vi "Window_plot.vi"() -> ()   [LabVIEW 2022 SP3]
doc: "This window has the capability to visualize and analyze the graphs of the stored signals from the Main_menu."
uses:
  <vilib>/Waveform/WDTOps.llb/WDT Get Waveform Subset DBL.vi
panel:
  in  "Slide Offset":u32(slide) scale=0.0..10.0
  in  "Select offset":string(combo)
  out "Waveform Graph":waveform(dbl)[](graph) caption="Waveform Graph 2"
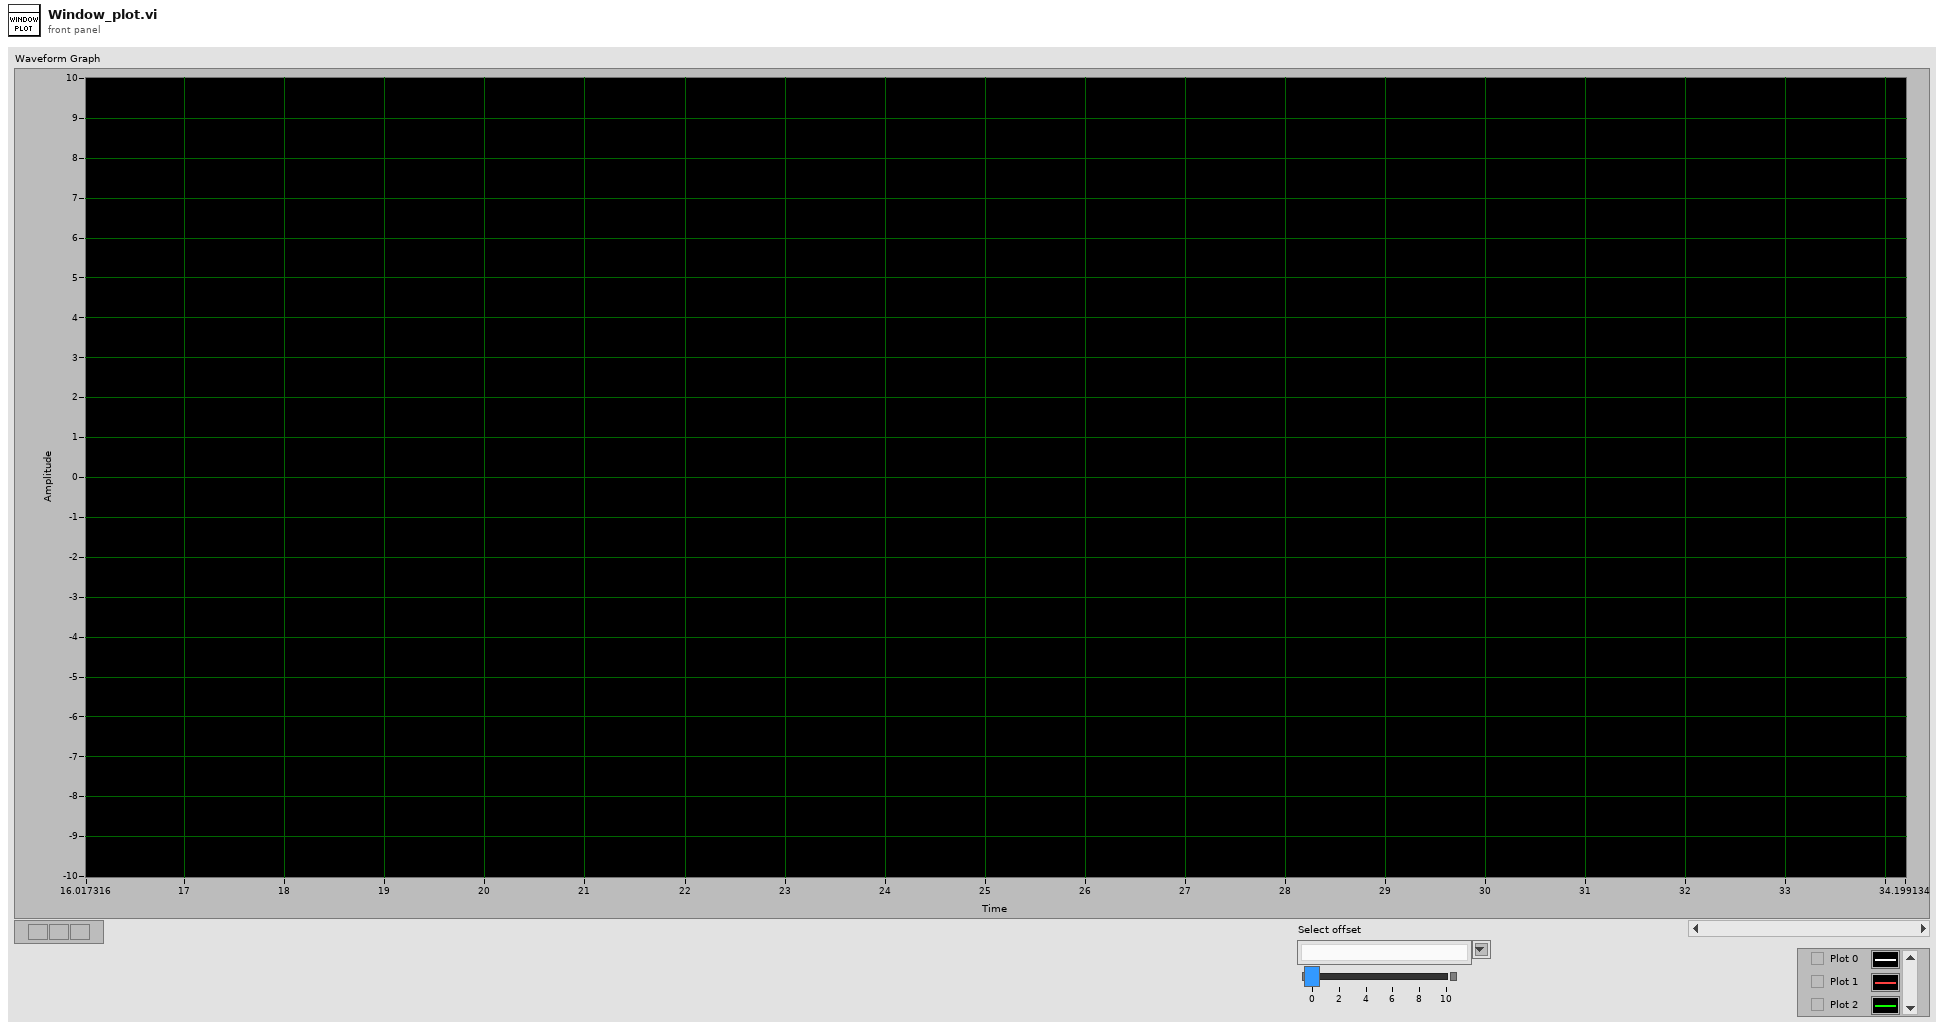
[diagram p1: front panel]
types:
  T1 = cluster{"Mode signal_Global":refnum<vi>, "Trace name":refnum<vi>, "Execution:State":refnum<vi>, "message":refnum<vi>, "Filename":refnum<vi>, "Closed w":refnum<vi>, "total \nrefresh time":refnum<vi>, "Mode signal_Global 2":string, "Filename 2":string, "Execution:State 2":enum32{"Bad", "Idle", "Run top level", "Running"}, "message 2":string, "Trace name 2":string, "total \nrefresh time 2":i32, "refresh time 2":i32, "Continous":bool}
  T2 = cluster{"plot Names":string[], "Waveforms arrays":waveform(dbl)[], "signals_HW":string[][], "Waveforms arrays csv":waveform(dbl)[], "signals_csv":string[], "Signals_name":string[], "Mode_signal_conf":u8, "Request_plots_array":cluster{string, waveform(dbl)}[], "time out":i32, " global r time":u32, "Refresh time":u32, "Local Mode":enum32{"Resume", "Hold"}}
  T3 = enum32{"Invalid", "Standard", "Closed", "Hidden", "Minimized", "Maximized"}
  T4 = enum32{"Bad", "Idle", "Run top level", "Running"}
  T5 = cluster{"plot Names":string[], "Waveforms arrays":waveform(dbl)[], "signals_HW":string[][], "Waveforms arrays csv":waveform(dbl)[], "signals_csv":string[], "Signals_name":string[], "Mode_signal_conf":u8, "Request_plots_array":cluster{string, "Waveform":waveform(dbl)}[], "time out":i32, " global r time":u32, "Refresh time":u32, "Local Mode":enum32{"Resume", "Hold"}}
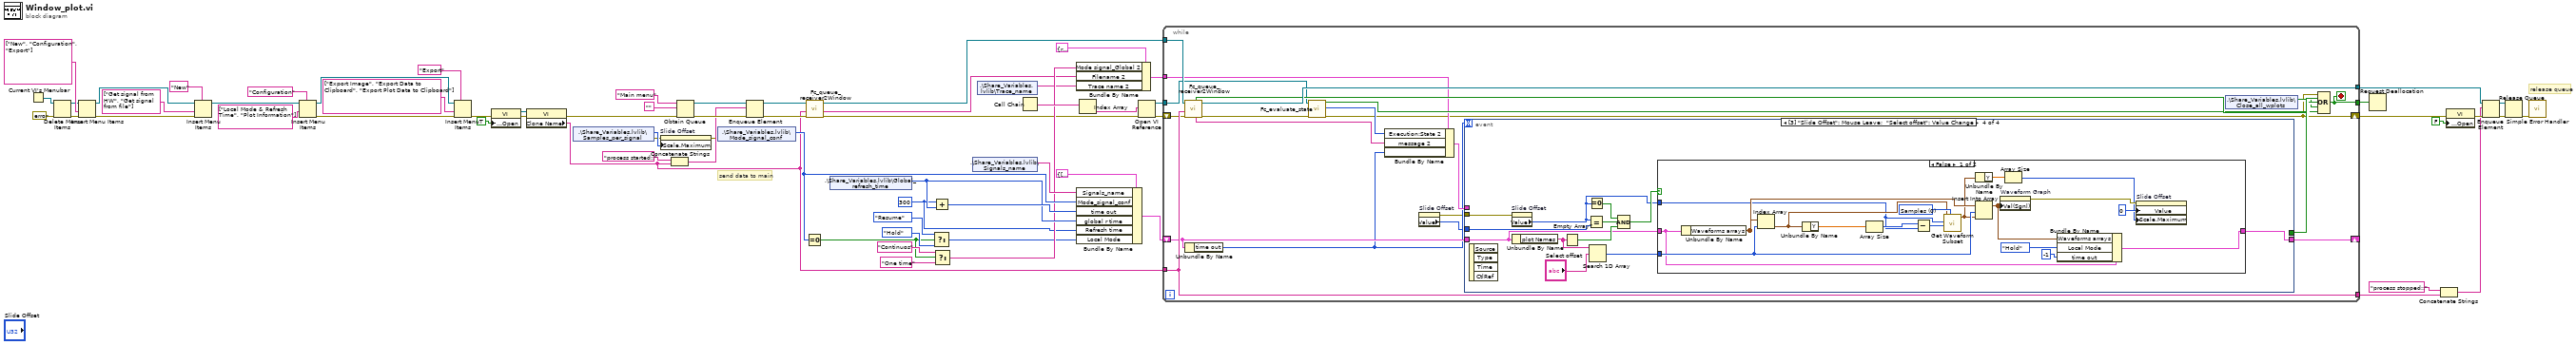
[diagram p0: block diagram]
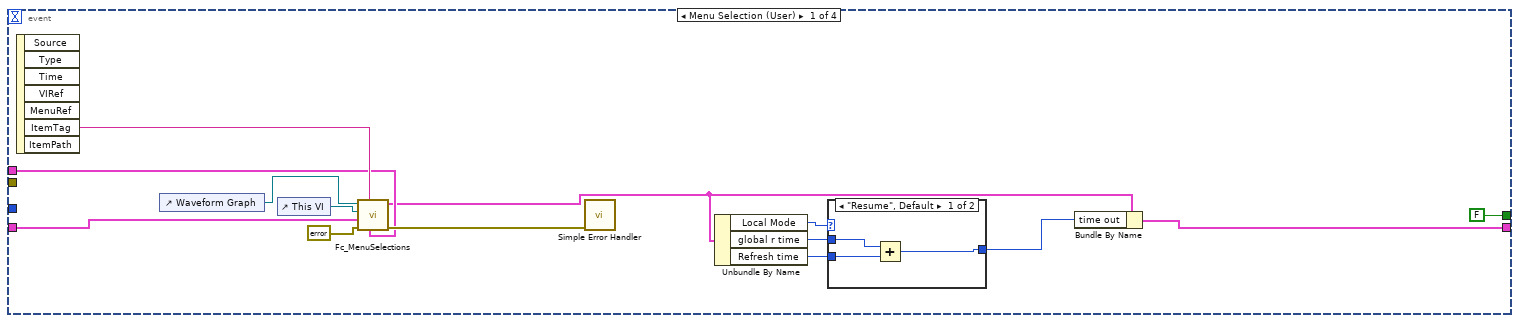
[diagram p2: hidden frame]
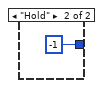
[diagram p3: hidden frame]
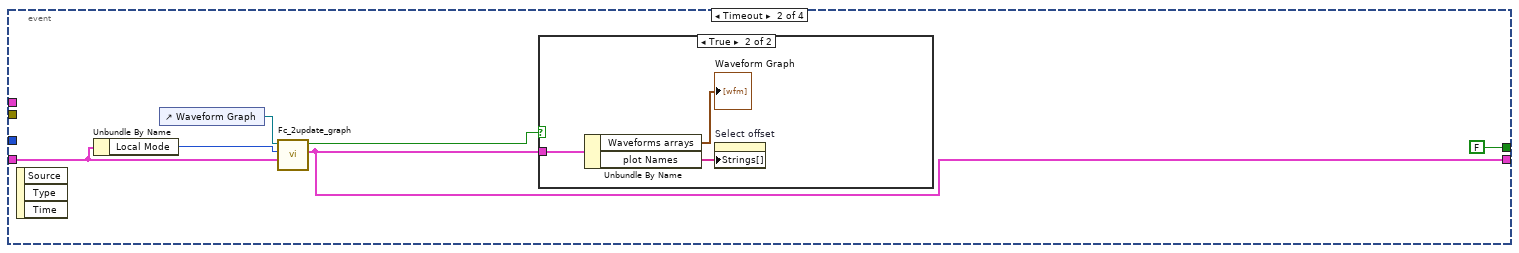
[diagram p4: hidden frame]
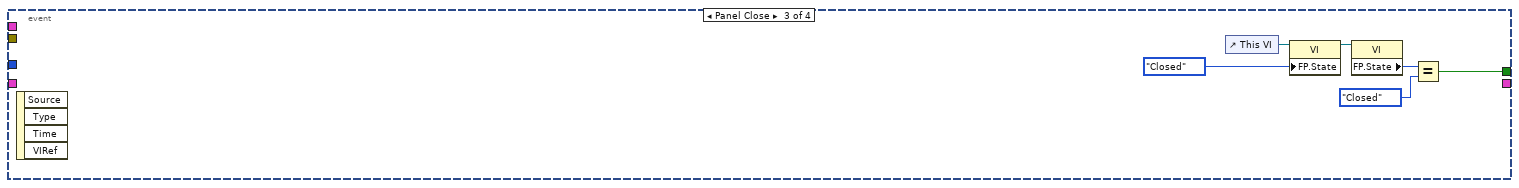
[diagram p6: hidden frame]
diagram:
  w32 = u32 300 ("Refresh time")
  # "send data to main"
  # "release queue"
  n1 = Current VI's Menubar() -> (w20:refnum<k9>)
  n2 = Delete Menu Items(6:errorcluster {"status"=FALSE, "code"=0, "source"=""} ("error in (no error)"), 9:w20) -> (0:w19:errorcluster, 3:w18:refnum<k9>)  [unwired: 2 in]
  n3 = Insert Menu Items(6:w19, 7:string[] ["New", "Configuration", "Export"], 9:w18) -> (0:w25:errorcluster, 3:w24:refnum<k9>)  [unwired: 3 in, 1 out]
  n4 = Insert Menu Items(5:"New", 6:w25, 7:string[] ["Get signal from HW", "Get signal from file"], 9:w24) -> (3:w13:refnum<k9>)  [unwired: 2 in, 2 out]
  n5 = Insert Menu Items(5:"Configuration" ("menu tag"), 7:string[] ["Local Mode & Refresh Time", "Plot Information"] ("item tags"), 9:w13) -> (0:w9:errorcluster, 3:w12:refnum<k9>)  [unwired: 3 in, 1 out]
  n6 = Insert Menu Items(5:"Export" ("menu tag"), 6:w9, 7:string[] ["Export Image", "Export Data to Clipboard", "Export Plot Data to Clipboard"], 9:w12) -> (0:w26:errorcluster)  [unwired: 2 in, 2 out]
  n7 = property class="VI"(error in=w26, "Front Panel.Open"=TRUE ("Front Panel Window:Open")) -> (reference out=w52:refnum<vi>, error out=w62:errorcluster)  [unwired: 1 in]
  n8 = property class="VI"(reference=w52, error in=w62) -> (error out=w45:errorcluster, "Clone Name"=w35:string)  [unwired: 1 out]
  n9 = shared-variable ".\\Share_Variables.lvlib\\Samples_per_signal"() -> (w4:u32, error out=w3:errorcluster)  [unwired: 1 in]
  n10 = property on="Slide Offset" class="Slide (strict)"(error in=w3, "Scale.Maximum"=w4) -> (error out=w1:errorcluster)  [unwired: 1 in, 1 out]
  n11 = Concatenate Strings("process started::" ("name (unnamed)"), w35) -> (w63:string)
  n12 = Obtain Queue(name (unnamed)="Main menu", element data type="", error in (no error)=w45) -> (queue out=w65:refnum<queue>, error out=w64:errorcluster)  [unwired: 2 in, 1 out]
  n13 = shared-variable ".\\Share_Variables.lvlib\\Mode_signal_conf"(error in=w1) -> (w46:u8)  [unwired: 1 out]
  n14 = Enqueue Element(queue=w65, element=w63, error in (no error)=w64) -> (queue out=w38:refnum<queue>, error out=w36:errorcluster)  [unwired: 1 in, 1 out]
  n15 = Equal To 0?(x=w46) -> (x = 0?=w6:bool)
  n16 = call "Fc_queue_receiver2Window.vi"("error in (no error)"=w36, "Clone Name"=w35, "Queue in"=w38) -> ("error out"=w2:errorcluster, "Filename"=w33:string, "Queue out"=w37:refnum<queue>)  [unwired: 4 in, 2 out]
  n17 = shared-variable ".\\Share_Variables.lvlib\\Global_refresh_time"() -> (w41:u16)  [unwired: 1 in, 1 out]
  n18 = Select(t=enum32{"Resume", "Hold"}."Resume" ("Local Mode"), s=w6, f=enum32{"Resume", "Hold"}."Hold" ("Local Mode")) -> (s? t:f=w30:enum32{"Resume", "Hold"})
  n19 = Add(x=w32, y=w41) -> (x+y=w42:u32)
  n20 = Select(t="Continuos", s=w6, f="One time") -> (s? t:f=w34:string)
  n21 = shared-variable ".\\Share_Variables.lvlib\\Signals_name"() -> (w47:string[])  [unwired: 1 in, 1 out]
  n22 = shared-variable ".\\Share_Variables.lvlib\\Trace_name"() -> (w31:string)  [unwired: 1 in, 1 out]
  n23 = Call Chain() -> (call chain=w51:string[])
  n24 = Bundle By Name(cluster=T1 {"Mode signal_Global"=refnum, "Trace name"=refnum, "Execution:State"=refnum, "message"=refnum, "Filename"=refnum, "Closed w"=refnum, "total \nrefresh time"=refnum, "Mode signal_Global 2"="", "Filename 2"="", "Execution:State 2"=enum."Idle", "message 2"="", "Trace name 2"="", "total \nrefresh time 2"=0, "refresh time 2"=0, "Continous"=TRUE}, "Mode signal_Global 2"=w34, "Filename 2"=w33, "Trace name 2"=w31) -> (w40:T1)
  n25 = Bundle By Name(cluster=T2 {"plot Names"=[], "Waveforms arrays"=[], "signals_HW"=[], "Waveforms arrays csv"=[], "signals_csv"=[], "Signals_name"=[], "Mode_signal_conf"=0, "Request_plots_array"=[], "time out"=300, " global r time"=0, "Refresh time"=0, "Local Mode"=enum."Resume"}, "Signals_name"=w47, "Mode_signal_conf"=w46, "time out"=w42, "global r time"=w41, "Refresh time"=w32, "Local Mode"=w30) -> (w48:T2)
  n26 = Index Array(array=w51) -> (element=w50:string)  [unwired: 1 in]
  n27 = Open VI Reference(vi path=w50, error in (no error)=w2) -> (vi reference=w49:refnum<vi>, error out=w28:errorcluster)  [unwired: 4 in]
  n28 = while {
    tunnel: w37 -> [w89]
    tunnel: [w88] -> w61
    shift-right: [w71] -> w56
    shift-left: w28 -> [w78]
    tunnel: [w83] -> w54
    tunnel: w49 -> [w81]
    tunnel: w35 -> [w83]
    shift-right: [w84] -> _
    shift-left: w48 -> [w82]
    tunnel: [w80] -> w44
    tunnel: w40 -> [w77]
    stop <- w80 stop-if-true
    n29 = call "Fc_queue_receiver2Window.vi"("error in (no error)"=w78, "Clone Name"=w83, "Queue in"=w89) -> ("error out"=w72:errorcluster, "Queue out"=w88:refnum<queue>, "message"=w74:string, "Stop"=w86:bool)  [unwired: 4 in, 1 out]
    n30 = Unbundle By Name(w82) -> ("time out"=w73:i32)
    n31 = call "Fc_evaluate_state.vi"("error in (no error)"=w72, "VI in"=w81) -> ("error out"=w71:errorcluster, "Exec.State"=w76:T4, "Status out"=w79:bool)  [unwired: 7 in]
    n32 = Bundle By Name(cluster=w77, "Execution:State 2"=w76, "message 2"=w74, "total \nrefresh time 2"=w73) -> (w75:T1)
    n33 = property on="Slide Offset" class="Slide (strict)"() -> (error out=w70:errorcluster, "Value"=w69:u32)  [unwired: 2 in, 1 out]
    n34 = event shown="[3] \"Slide Offset\": Mouse Leave;  \"Select offset\": Value Change" {
      selector: _ -> [_ _ _ _]
      dyn-events: _ -> [_ _ _ _]
      timeout: w73 -> [_ _ _ _]
      tunnel: [FALSE FALSE w120 _] -> w87
      tunnel: [w90 w108 _ w123] -> w84
      tunnel: w82 -> [w95 w110 _ w126]
      tunnel: w75 -> [w97 _ _ _]
      tunnel: w70 -> [_ _ _ w134]
      tunnel: w69 -> [_ _ _ w132]
      event Menu Selection (User) {
        n35 = event-data() -> ("ItemTag"=w103:string)  [unwired: 1 in, 6 out]
        n36 = control-ref of="Waveform Graph"() -> (w99:refnum<vi>)
        n37 = control-ref of="This VI"() -> (w98:refnum<vi>)
        n38 = call "Fc_MenuSelections.vi"("Cluster References"=w97, "ItemTag"=w103, "error in (no error)"=errorcluster {"status"=FALSE, "code"=0, "source"=""}, "Cluster in"=w95, "VI caller"=w98, "WaveformGraph in"=w99) -> ("error out"=w101:errorcluster, "Cluster out"=w91:T5)  [unwired: 4 in]
        n39 = call <vilib>:"Simple Error Handler.vi"("error in (no error)"=w101) -> ()  [unwired: 4 in, 5 out]
        n40 = Unbundle By Name(w91) -> ("Local Mode"=w94:enum32{"Resume", "Hold"}, "global r time"=w93:u32, "Refresh time"=w92:u32)
        n41 = case shown="\"Resume\", Default" w94 {
          tunnel: [w104 -1 ("time out")] -> w96
          tunnel: w93 -> [w106 _]
          tunnel: w92 -> [w105 _]
          frame "Resume", Default {
            n42 = Add(x=w106, y=w105) -> (x+y=w104:u32)
          }
          frame "Hold" {
          }
        }
        n43 = Bundle By Name(cluster=w91, "time out"=w96) -> (w90:T5)
      }
      event Timeout {
        n44 = event-data() -> ()  [unwired: 1 in, 3 out]
        n45 = Unbundle By Name(w110) -> ("Local Mode"=w109:enum32{"Resume", "Hold"})
        n46 = control-ref of="Waveform Graph"() -> (w111:refnum<vi>)
        n47 = call "Fc_2update_graph.vi"("Cluster in"=w110, "Local Mode"=w109, "WaveformGraph in"=w111) -> ("Cluster in 2"=w108:T5, "Update Waveform Graph"=w112:bool)  [unwired: 7 in]
        n48 = case shown="True" w112 {
          tunnel: w108 -> [_ w115]
          frame False {
          }
          frame True {
            n49 = Unbundle By Name(w115) -> ("Waveforms arrays"=→"Waveform Graph":waveform(dbl)[], "plot Names"=w114:string[])
            n50 = property on="Select offset" class="CmbBox"("Strings[]"=w114) -> ()  [unwired: 2 in, 2 out]
          }
        }
      }
      event Panel Close {
        n51 = event-data() -> ()  [unwired: 1 in, 4 out]
        n52 = control-ref of="This VI"() -> (w119:refnum<vi>)
        n53 = property class="VI"(reference=w119, "FP.State"=T3."Closed" ("Front Panel Window:State")) -> (reference out=w117:refnum<vi>)  [unwired: 1 in, 1 out]
        n54 = property class="VI"(reference=w117) -> ("FP.State"=w121:T3)  [unwired: 1 in, 2 out]
        n55 = Equal?(x=w121, y=T3."Closed" ("Front Panel Window:State")) -> (x = y?=w120:bool)
      }
      event "Slide Offset": Mouse Leave; "Select offset": Value Change {
        n56 = event-data() -> ()  [unwired: 1 in, 4 out]
        n57 = property on="Slide Offset" class="Slide (strict)"(error in=w134) -> ("Value"=w124:u32)  [unwired: 1 in, 2 out]
        n58 = Unbundle By Name(w126) -> ("plot Names"=w127:string[])
        n59 = Empty Array?(array=w127) -> (empty?=w129:bool)
        n60 = Equal?(x=w124, y=w132) -> (x = y?=w130:bool)
        n61 = Equal To 0?(x=w124) -> (x = 0?=w131:bool)
        n62 = Search 1D Array(1D array=w127, element="Select offset") -> (index of element=w125:i32)  [unwired: 1 in]
        n63 = Compound Arithmetic op=AND(w131, w130, w129) -> (w128:bool)
        n64 = case shown="False" w128 {
          tunnel: w126 -> [w139 w153]
          tunnel: w125 -> [w147 _]
          tunnel: w124 -> [w145 _]
          tunnel: [w138 w153] -> w123
          frame False {
            w151 = u16 0 items=["Samples", "Relative Time"] ("start/duration format")
            n65 = Unbundle By Name(w139) -> ("Waveforms arrays"=w148:waveform(dbl)[])
            n66 = Index Array(array=w148, index=w147) -> (element=w150:waveform(dbl))
            n67 = Unbundle By Name(w150) -> ("Y"=w152:dbl[])
            n68 = Array Size(array=w152) -> (size(s)=w149:i32)
            n69 = Subtract(x=w149, y=w145) -> (x-y=w146:u32)
            n70 = call-poly <vilib>:"Get Waveform Subset.vi"("start/duration format"=w151, "duration"=w146, "start samples/time"=w145, "waveform in"=w150) -> ("waveform out"=w142:waveform(dbl))  [unwired: 2 in, 3 out]
            n71 = Unbundle By Name(w142) -> ("Y"=w141:dbl[])
            n72 = Insert Into Array(array=w148, index=w147, new element=w142) -> (w137:waveform(dbl)[])
            n73 = property on="Waveform Graph" class="WFGraph (strict)"("Val(Sgnl)"=w137) -> (error out=w144:errorcluster)  [unwired: 2 in, 1 out]
            n74 = Array Size(array=w141) -> (size(s)=w140:i32)
            n75 = Bundle By Name(cluster=w139, "Waveforms arrays"=w137, "Local Mode"=enum32{"Resume", "Hold"}."Hold", "time out"=-1) -> (w138:T2)
            n76 = property on="Slide Offset" class="Slide (strict)"(error in=w144, "Value"=u32 0 ("Slide Offset"), "Scale.Maximum"=w140) -> ()  [unwired: 1 in, 2 out]
          }
          frame True {
          }
        }
      }
    }
    n77 = shared-variable ".\\Share_Variables.lvlib\\Close_all_wplots"() -> (w85:bool)  [unwired: 1 in, 1 out]
    n78 = Compound Arithmetic op=OR(w71, w87, w86, w85, w79) -> (w80:bool)
  }
  n79 = Request Deallocation(w44) -> ()
  n80 = Concatenate Strings("process stopped::" ("string"), w54) -> (w53:string)
  n81 = property class="VI"(error in=w56, "Front Panel.Open"=FALSE ("Front Panel Window:Open")) -> (error out=w58:errorcluster)  [unwired: 1 in, 1 out]
  n82 = Enqueue Element(queue=w61, element=w53, error in (no error)=w58) -> (queue out=w60:refnum<queue>, error out=w59:errorcluster)  [unwired: 1 in, 1 out]
  n83 = Release Queue(queue=w60, error in (no error)=w59) -> (error out=w29:errorcluster)  [unwired: 1 in, 2 out]
  n84 = call <vilib>:"Simple Error Handler.vi"("error in (no error)"=w29) -> ()  [unwired: 4 in, 5 out]
